vi "App - analyze RUS V6.vi"() -> ()   [LabVIEW 2015] (continued)
Field(T) "=0.0}, {"temperature"=205.505, "temperature str"="205.50500", "file path"=path "D:/Data/Ultrasound/LSCO/LSCO22__130814c/5_Cooling_2nd_try/September_2014/091614/205.50500K_500_2500_2.10000V_0.00000T_Sep16-2014__13-51-53_001_091614.bin", "last mod"=timestamp(3493734713 s since 1904-01-01), "file name str"="D:\\Data\\Ultrasound\\LSCO\\LSCO22__130814c\\5_Cooling_2nd_try\\September_2014\\091614\\205.50500K_500_2500_2.10000V_0.00000T_Sep16-2014__13-51-53_001_091614.bin", "mod time(min)"=58228911.88333333, "file format"=enum."binary", "power(V)"=2.1, "Magn Field(T) "=0.0}, {"temperature"=205.23, "temperature str"="205.23000", "file path"=path "D:/Data/Ultrasound/LSCO/LSCO22__130814c/5_Cooling_2nd_try/September_2014/091614/205.23000K_500_2500_2.10000V_0.00000T_Sep16-2014__13-53-13_001_091614.bin", "last mod"=timestamp(3493734793 s since 1904-01-01), "file name str"="D:\\Data\\Ultrasound\\LSCO\\LSCO22__130814c\\5_Cooling_2nd_try\\September_2014\\091614\\205.23000K_500_2500_2.10000V_0.00000T_Sep16-2014__13-53-13_001_091614.bin", "mod time(min)"=58228913.21666667, "file format"=enum."binary", "power(V)"=2.1, "Magn Field(T) "=0.0}, {"temperature"=204.949, "temperature str"="204.94900", "file path"=path "D:/Data/Ultrasound/LSCO/LSCO22__130814c/5_Cooling_2nd_try/September_2014/091614/204.94900K_500_2500_2.10000V_0.00000T_Sep16-2014__13-54-32_001_091614.bin", "last mod"=timestamp(3493734872 s since 1904-01-01), "file name str"="D:\\Data\\Ultrasound\\LSCO\\LSCO22__130814c\\5_Cooling_2nd_try\\September_2014\\091614\\204.94900K_500_2500_2.10000V_0.00000T_Sep16-2014__13-54-32_001_091614.bin", "mod time(min)"=58228914.53333333, "file format"=enum."binary", "power(V)"=2.1, "Magn Field(T) "=0.0}, {"temperature"=204.683, "temperature str"="204.68300", "file path"=path "D:/Data/Ultrasound/LSCO/LSCO22__130814c/5_Cooling_2nd_try/September_2014/091614/204.68300K_500_2500_2.10000V_0.00000T_Sep16-2014__13-55-52_001_091614.bin", "last mod"=timestamp(3493734952 s since 1904-01-01), "file name str"="D:\\Data\\Ultrasound\\LSCO\\LSCO22__130814c\\5_Cooling_2nd_try\\September_2014\\091614\\204.68300K_500_2500_2.10000V_0.00000T_Sep16-2014__13-55-52_001_091614.bin", "mod time(min)"=58228915.86666667, "file format"=enum."binary", "power(V)"=2.1, "Magn Field(T) "=0.0}, {"temperature"=204.406, "temperature str"="204.40600", "file path"=path "D:/Data/Ultrasound/LSCO/LSCO22__130814c/5_Cooling_2nd_try/September_2014/091614/204.40600K_500_2500_2.10000V_0.00000T_Sep16-2014__13-57-11_001_091614.bin", "last mod"=timestamp(3493735031 s since 1904-01-01), "file name str"="D:\\Data\\Ultrasound\\LSCO\\LSCO22__130814c\\5_Cooling_2nd_try\\September_2014\\091614\\204.40600K_500_2500_2.10000V_0.00000T_Sep16-2014__13-57-11_001_091614.bin", "mod time(min)"=58228917.18333333, "file format"=enum."binary", "power(V)"=2.1, "Magn Field(T) "=0.0}, {"temperature"=204.135, "temperature str"="204.13500", "file path"=path "D:/Data/Ultrasound/LSCO/LSCO22__130814c/5_Cooling_2nd_try/September_2014/091614/204.13500K_500_2500_2.10000V_0.00000T_Sep16-2014__13-58-30_001_091614.bin", "last mod"=timestamp(3493735110 s since 1904-01-01), "file name str"="D:\\Data\\Ultrasound\\LSCO\\LSCO22__130814c\\5_Cooling_2nd_try\\September_2014\\091614\\204.13500K_500_2500_2.10000V_0.00000T_Sep16-2014__13-58-30_001_091614.bin", "mod time(min)"=58228918.5, "file format"=enum."binary", "power(V)"=2.1, "Magn Field(T) "=0.0}, {"temperature"=203.855, "temperature str"="203.85500", "file path"=path "D:/Data/Ultrasound/LSCO/LSCO22__130814c/5_Cooling_2nd_try/September_2014/091614/203.85500K_500_2500_2.10000V_0.00000T_Sep16-2014__13-59-50_001_091614.bin", "last mod"=timestamp(3493735190 s since 1904-01-01), "file name str"="D:\\Data\\Ultrasound\\LSCO\\LSCO22__130814c\\5_Cooling_2nd_try\\September_2014\\091614\\203.85500K_500_2500_2.10000V_0.00000T_Sep16-2014__13-59-50_001_091614.bin", "mod time(min)"=58228919.833333336, "file format"=enum."binary", "power(V)"=2.1, "Magn Field(T) "=0.0}, {"temperature"=203.577, "temperature str"="203.57700", "file path"=path "D:/Data/Ultrasound/LSCO/LSCO22__130814c/5_Cooling_2nd_try/September_2014/091614/203.57700K_500_2500_2.10000V_0.00000T_Sep16-2014__14-01-09_001_091614.bin", "last mod"=timestamp(3493735269 s since 1904-01-01), "file name str"="D:\\Data\\Ultrasound\\LSCO\\LSCO22__130814c\\5_Cooling_2nd_try\\September_2014\\091614\\203.57700K_500_2500_2.10000V_0.00000T_Sep16-2014__14-01-09_001_091614.bin", "mod time(min)"=58228921.15, "file format"=enum."binary", "power(V)"=2.1, "Magn Field(T) "=0.0}, {"temperature"=203.306, "temperature str"="203.30600", "file path"=path "D:/Data/Ultrasound/LSCO/LSCO22__130814c/5_Cooling_2nd_try/September_2014/091614/203.30600K_500_2500_2.10000V_0.00000T_Sep16-2014__14-02-28_001_091614.bin", "last mod"=timestamp(3493735348 s since 1904-01-01), "file name str"="D:\\Data\\Ultrasound\\LSCO\\LSCO22__130814c\\5_Cooling_2nd_try\\September_2014\\091614\\203.30600K_500_2500_2.10000V_0.00000T_Sep16-2014__14-02-28_001_091614.bin", "mod time(min)"=58228922.46666667, "file format"=enum."binary", "power(V)"=2.1, "Magn Field(T) "=0.0}, {"temperature"=203.002, "temperature str"="203.00200", "file path"=path "D:/Data/Ultrasound/LSCO/LSCO22__130814c/5_Cooling_2nd_try/September_2014/091614/203.00200K_500_2500_2.10000V_0.00000T_Sep16-2014__14-03-54_001_091614.bin", "last mod"=timestamp(3493735434 s since 1904-01-01), "file name str"="D:\\Data\\Ultrasound\\LSCO\\LSCO22__130814c\\5_Cooling_2nd_try\\September_2014\\091614\\203.00200K_500_2500_2.10000V_0.00000T_Sep16-2014__14-03-54_001_091614.bin", "mod time(min)"=58228923.9, "file format"=enum."binary", "power(V)"=2.1, "Magn Field(T) "=0.0}, {"temperature"=202.734, "temperature str"="202.73400", "file path"=path "D:/Data/Ultrasound/LSCO/LSCO22__130814c/5_Cooling_2nd_try/September_2014/091614/202.73400K_500_2500_2.10000V_0.00000T_Sep16-2014__14-05-13_001_091614.bin", "last mod"=timestamp(3493735513 s since 1904-01-01), "file name str"="D:\\Data\\Ultrasound\\LSCO\\LSCO22__130814c\\5_Cooling_2nd_try\\September_2014\\091614\\202.73400K_500_2500_2.10000V_0.00000T_Sep16-2014__14-05-13_001_091614.bin", "mod time(min)"=58228925.21666667, "file format"=enum."binary", "power(V)"=2.1, "Magn Field(T) "=0.0}, {"temperature"=202.449, "temperature str"="202.44900", "file path"=path "D:/Data/Ultrasound/LSCO/LSCO22__130814c/5_Cooling_2nd_try/September_2014/091614/202.44900K_500_2500_2.10000V_0.00000T_Sep16-2014__14-06-32_001_091614.bin", "last mod"=timestamp(3493735592 s since 1904-01-01), "file name str"="D:\\Data\\Ultrasound\\LSCO\\LSCO22__130814c\\5_Cooling_2nd_try\\September_2014\\091614\\202.44900K_500_2500_2.10000V_0.00000T_Sep16-2014__14-06-32_001_091614.bin", "mod time(min)"=58228926.53333333, "file format"=enum."binary", "power(V)"=2.1, "Magn Field(T) "=0.0}, {"temperature"=202.176, "temperature str"="202.17600", "file path"=path "D:/Data/Ultrasound/LSCO/LSCO22__130814c/5_Cooling_2nd_try/September_2014/091614/202.17600K_500_2500_2.10000V_0.00000T_Sep16-2014__14-07-52_001_091614.bin", "last mod"=timestamp(3493735672 s since 1904-01-01), "file name str"="D:\\Data\\Ultrasound\\LSCO\\LSCO22__130814c\\5_Cooling_2nd_try\\September_2014\\091614\\202.17600K_500_2500_2.10000V_0.00000T_Sep16-2014__14-07-52_001_091614.bin", "mod time(min)"=58228927.86666667, "file format"=enum."binary", "power(V)"=2.1, "Magn Field(T) "=0.0}, {"temperature"=201.892, "temperature str"="201.89200", "file path"=path "D:/Data/Ultrasound/LSCO/LSCO22__130814c/5_Cooling_2nd_try/September_2014/091614/201.89200K_500_2500_2.10000V_0.00000T_Sep16-2014__14-09-11_001_091614.bin", "last mod"=timestamp(3493735751 s since 1904-01-01), "file name str"="D:\\Data\\Ultrasound\\LSCO\\LSCO22__130814c\\5_Cooling_2nd_try\\September_2014\\091614\\201.89200K_500_2500_2.10000V_0.00000T_Sep16-2014__14-09-11_001_091614.bin", "mod time(min)"=58228929.18333333, "file format"=enum."binary", "power(V)"=2.1, "Magn Field(T) "=0.0}, {"temperature"=201.608, "temperature str"="201.60800", "file path"=path "D:/Data/Ultrasound/LSCO/LSCO22__130814c/5_Cooling_2nd_try/September_2014/091614/201.60800K_500_2500_2.10000V_0.00000T_Sep16-2014__14-10-30_001_091614.bin", "last mod"=timestamp(3493735830 s since 1904-01-01), "file name str"="D:\\Data\\Ultrasound\\LSCO\\LSCO22__130814c\\5_Cooling_2nd_try\\September_2014\\091614\\201.60800K_500_2500_2.10000V_0.00000T_Sep16-2014__14-10-30_001_091614.bin", "mod time(min)"=58228930.5, "file format"=enum."binary", "power(V)"=2.1, "Magn Field(T) "=0.0}, {"temperature"=201.335, "temperature str"="201.33500", "file path"=path "D:/Data/Ultrasound/LSCO/LSCO22__130814c/5_Cooling_2nd_try/September_2014/091614/201.33500K_500_2500_2.10000V_0.00000T_Sep16-2014__14-11-50_001_091614.bin", "last mod"=timestamp(3493735910 s since 1904-01-01), "file name str"="D:\\Data\\Ultrasound\\LSCO\\LSCO22__130814c\\5_Cooling_2nd_try\\September_2014\\091614\\201.33500K_500_2500_2.10000V_0.00000T_Sep16-2014__14-11-50_001_091614.bin", "mod time(min)"=58228931.833333336, "file format"=enum."binary", "power(V)"=2.1, "Magn Field(T) "=0.0}, {"temperature"=201.049, "temperature str"="201.04900", "file path"=path "D:/Data/Ultrasound/LSCO/LSCO22__130814c/5_Cooling_2nd_try/September_2014/091614/201.04900K_500_2500_2.10000V_0.00000T_Sep16-2014__14-13-09_001_091614.bin", "last mod"=timestamp(3493735989 s since 1904-01-01), "file name str"="D:\\Data\\Ultrasound\\LSCO\\LSCO22__130814c\\5_Cooling_2nd_try\\September_2014\\091614\\201.04900K_500_2500_2.10000V_0.00000T_Sep16-2014__14-13-09_001_091614.bin", "mod time(min)"=58228933.15, "file format"=enum."binary", "power(V)"=2.1, "Magn Field(T) "=0.0}, {"temperature"=200.772, "temperature str"="200.77200", "file path"=path "D:/Data/Ultrasound/LSCO/LSCO22__130814c/5_Cooling_2nd_try/September_2014/091614/200.77200K_500_2500_2.10000V_0.00000T_Sep16-2014__14-14-29_001_091614.bin", "last mod"=timestamp(3493736069 s since 1904-01-01), "file name str"="D:\\Data\\Ultrasound\\LSCO\\LSCO22__130814c\\5_Cooling_2nd_try\\September_2014\\091614\\200.77200K_500_2500_2.10000V_0.00000T_Sep16-2014__14-14-29_001_091614.bin", "mod time(min)"=58228934.483333334, "file format"=enum."binary", "power(V)"=2.1, "Magn Field(T) "=0.0}, {"temperature"=200.485, "temperature str"="200.48500", "file path"=path "D:/Data/Ultrasound/LSCO/LSCO22__130814c/5_Cooling_2nd_try/September_2014/091614/200.48500K_500_2500_2.10000V_0.00000T_Sep16-2014__14-15-48_001_091614.bin", "last mod"=timestamp(3493736148 s since 1904-01-01), "file name str"="D:\\Data\\Ultrasound\\LSCO\\LSCO22__130814c\\5_Cooling_2nd_try\\September_2014\\091614\\200.48500K_500_2500_2.10000V_0.00000T_Sep16-2014__14-15-48_001_091614.bin", "mod time(min)"=58228935.8, "file format"=enum."binary", "power(V)"=2.1, "Magn Field(T) "=0.0}, {"temperature"=200.196, "temperature str"="200.19600", "file path"=path "D:/Data/Ultrasound/LSCO/LSCO22__130814c/5_Cooling_2nd_try/September_2014/091614/200.19600K_500_2500_2.10000V_0.00000T_Sep16-2014__14-17-07_001_091614.bin", "last mod"=timestamp(3493736227 s since 1904-01-01), "file name str"="D:\\Data\\Ultrasound\\LSCO\\LSCO22__130814c\\5_Cooling_2nd_try\\September_2014\\091614\\200.19600K_500_2500_2.10000V_0.00000T_Sep16-2014__14-17-07_001_091614.bin", "mod time(min)"=58228937.11666667, "file format"=enum."binary", "power(V)"=2.1, "Magn Field(T) "=0.0}, {"temperature"=199.92, "temperature str"="199.92000", "file path"=path "D:/Data/Ultrasound/LSCO/LSCO22__130814c/5_Cooling_2nd_try/September_2014/091614/199.92000K_500_2500_2.10000V_0.00000T_Sep16-2014__14-18-27_001_091614.bin", "last mod"=timestamp(3493736307 s since 1904-01-01), "file name str"="D:\\Data\\Ultrasound\\LSCO\\LSCO22__130814c\\5_Cooling_2nd_try\\September_2014\\091614\\199.92000K_500_2500_2.10000V_0.00000T_Sep16-2014__14-18-27_001_091614.bin", "mod time(min)"=58228938.45, "file format"=enum."binary", "power(V)"=2.1, "Magn Field(T) "=0.0}, {"temperature"=199.633, "temperature str"="199.63300", "file path"=path "D:/Data/Ultrasound/LSCO/LSCO22__130814c/5_Cooling_2nd_try/September_2014/091614/199.63300K_500_2500_2.10000V_0.00000T_Sep16-2014__14-19-46_001_091614.bin", "last mod"=timestamp(3493736386 s since 1904-01-01), "file name str"="D:\\Data\\Ultrasound\\LSCO\\LSCO22__130814c\\5_Cooling_2nd_try\\September_2014\\091614\\199.63300K_500_2500_2.10000V_0.00000T_Sep16-2014__14-19-46_001_091614.bin", "mod time(min)"=58228939.766666666, "file format"=enum."binary", "power(V)"=2.1, "Magn Field(T) "=0.0}, {"temperature"=199.352, "temperature str"="199.35200", "file path"=path "D:/Data/Ultrasound/LSCO/LSCO22__130814c/5_Cooling_2nd_try/September_2014/091614/199.35200K_500_2500_2.10000V_0.00000T_Sep16-2014__14-21-05_001_091614.bin", "last mod"=timestamp(3493736465 s since 1904-01-01), "file name str"="D:\\Data\\Ultrasound\\LSCO\\LSCO22__130814c\\5_Cooling_2nd_try\\September_2014\\091614\\199.35200K_500_2500_2.10000V_0.00000T_Sep16-2014__14-21-05_001_091614.bin", "mod time(min)"=58228941.083333336, "file format"=enum."binary", "power(V)"=2.1, "Magn Field(T) "=0.0}, {"temperature"=199.061, "temperature str"="199.06100", "file path"=path "D:/Data/Ultrasound/LSCO/LSCO22__130814c/5_Cooling_2nd_try/September_2014/091614/199.06100K_500_2500_2.10000V_0.00000T_Sep16-2014__14-22-25_001_091614.bin", "last mod"=timestamp(3493736545 s since 1904-01-01), "file name str"="D:\\Data\\Ultrasound\\LSCO\\LSCO22__130814c\\5_Cooling_2nd_try\\September_2014\\091614\\199.06100K_500_2500_2.10000V_0.00000T_Sep16-2014__14-22-25_001_091614.bin", "mod time(min)"=58228942.416666664, "file format"=enum."binary", "power(V)"=2.1, "Magn Field(T) "=0.0}, {"temperature"=198.769, "temperature str"="198.76900", "file path"=path "D:/Data/Ultrasound/LSCO/LSCO22__130814c/5_Cooling_2nd_try/September_2014/091614/198.76900K_500_2500_2.10000V_0.00000T_Sep16-2014__14-23-44_001_091614.bin", "last mod"=timestamp(3493736624 s since 1904-01-01), "file name str"="D:\\Data\\Ultrasound\\LSCO\\LSCO22__130814c\\5_Cooling_2nd_try\\September_2014\\091614\\198.76900K_500_2500_2.10000V_0.00000T_Sep16-2014__14-23-44_001_091614.bin", "mod time(min)"=58228943.733333334, "file format"=enum."binary", "power(V)"=2.1, "Magn Field(T) "=0.0}, {"temperature"=198.49, "temperature str"="198.49000", "file path"=path "D:/Data/Ultrasound/LSCO/LSCO22__130814c/5_Cooling_2nd_try/September_2014/091614/198.49000K_500_2500_2.10000V_0.00000T_Sep16-2014__14-25-04_001_091614.bin", "last mod"=timestamp(3493736704 s since 1904-01-01), "file name str"="D:\\Data\\Ultrasound\\LSCO\\LSCO22__130814c\\5_Cooling_2nd_try\\September_2014\\091614\\198.49000K_500_2500_2.10000V_0.00000T_Sep16-2014__14-25-04_001_091614.bin", "mod time(min)"=58228945.06666667, "file format"=enum."binary", "power(V)"=2.1, "Magn Field(T) "=0.0}, {"temperature"=198.198, "temperature str"="198.19800", "file path"=path "D:/Data/Ultrasound/LSCO/LSCO22__130814c/5_Cooling_2nd_try/September_2014/091614/198.19800K_500_2500_2.10000V_0.00000T_Sep16-2014__14-26-23_001_091614.bin", "last mod"=timestamp(3493736783 s since 1904-01-01), "file name str"="D:\\Data\\Ultrasound\\LSCO\\LSCO22__130814c\\5_Cooling_2nd_try\\September_2014\\091614\\198.19800K_500_2500_2.10000V_0.00000T_Sep16-2014__14-26-23_001_091614.bin", "mod time(min)"=58228946.38333333, "file format"=enum."binary", "power(V)"=2.1, "Magn Field(T) "=0.0}, {"temperature"=197.916, "temperature str"="197.91600", "file path"=path "D:/Data/Ultrasound/LSCO/LSCO22__130814c/5_Cooling_2nd_try/September_2014/091614/197.91600K_500_2500_2.10000V_0.00000T_Sep16-2014__14-27-42_001_091614.bin", "last mod"=timestamp(3493736862 s since 1904-01-01), "file name str"="D:\\Data\\Ultrasound\\LSCO\\LSCO22__130814c\\5_Cooling_2nd_try\\September_2014\\091614\\197.91600K_500_2500_2.10000V_0.00000T_Sep16-2014__14-27-42_001_091614.bin", "mod time(min)"=58228947.7, "file format"=enum."binary", "power(V)"=2.1, "Magn Field(T) "=0.0}, {"temperature"=197.62, "temperature str"="197.62000", "file path"=path "D:/Data/Ultrasound/LSCO/LSCO22__130814c/5_Cooling_2nd_try/September_2014/091614/197.62000K_500_2500_2.10000V_0.00000T_Sep16-2014__14-29-02_001_091614.bin", "last mod"=timestamp(3493736942 s since 1904-01-01), "file name str"="D:\\Data\\Ultrasound\\LSCO\\LSCO22__130814c\\5_Cooling_2nd_try\\September_2014\\091614\\197.62000K_500_2500_2.10000V_0.00000T_Sep16-2014__14-29-02_001_091614.bin", "mod time(min)"=58228949.03333333, "file format"=enum."binary", "power(V)"=2.1, "Magn Field(T) "=0.0}, {"temperature"=197.325, "temperature str"="197.32500", "file path"=path "D:/Data/Ultrasound/LSCO/LSCO22__130814c/5_Cooling_2nd_try/September_2014/091614/197.32500K_500_2500_2.10000V_0.00000T_Sep16-2014__14-30-21_001_091614.bin", "last mod"=timestamp(3493737021 s since 1904-01-01), "file name str"="D:\\Data\\Ultrasound\\LSCO\\LSCO22__130814c\\5_Cooling_2nd_try\\September_2014\\091614\\197.32500K_500_2500_2.10000V_0.00000T_Sep16-2014__14-30-21_001_091614.bin", "mod time(min)"=58228950.35, "file format"=enum."binary", "power(V)"=2.1, "Magn Field(T) "=0.0}, {"temperature"=197.042, "temperature str"="197.04200", "file path"=path "D:/Data/Ultrasound/LSCO/LSCO22__130814c/5_Cooling_2nd_try/September_2014/091614/197.04200K_500_2500_2.10000V_0.00000T_Sep16-2014__14-31-40_001_091614.bin", "last mod"=timestamp(3493737100 s since 1904-01-01), "file name str"="D:\\Data\\Ultrasound\\LSCO\\LSCO22__130814c\\5_Cooling_2nd_try\\September_2014\\091614\\197.04200K_500_2500_2.10000V_0.00000T_Sep16-2014__14-31-40_001_091614.bin", "mod time(min)"=58228951.666666664, "file format"=enum."binary", "power(V)"=2.1, "Magn Field(T) "=0.0}, {"temperature"=196.746, "temperature str"="196.74600", "file path"=path "D:/Data/Ultrasound/LSCO/LSCO22__130814c/5_Cooling_2nd_try/September_2014/091614/196.74600K_500_2500_2.10000V_0.00000T_Sep16-2014__14-33-00_001_091614.bin", "last mod"=timestamp(3493737180 s since 1904-01-01), "file name str"="D:\\Data\\Ultrasound\\LSCO\\LSCO22__130814c\\5_Cooling_2nd_try\\September_2014\\091614\\196.74600K_500_2500_2.10000V_0.00000T_Sep16-2014__14-33-00_001_091614.bin", "mod time(min)"=58228953.0, "file format"=enum."binary", "power(V)"=2.1, "Magn Field(T) "=0.0}, {"temperature"=196.459, "temperature str"="196.45900", "file path"=path "D:/Data/Ultrasound/LSCO/LSCO22__130814c/5_Cooling_2nd_try/September_2014/091614/196.45900K_500_2500_2.10000V_0.00000T_Sep16-2014__14-34-19_001_091614.bin", "last mod"=timestamp(3493737259 s since 1904-01-01), "file name str"="D:\\Data\\Ultrasound\\LSCO\\LSCO22__130814c\\5_Cooling_2nd_try\\September_2014\\091614\\196.45900K_500_2500_2.10000V_0.00000T_Sep16-2014__14-34-19_001_091614.bin", "mod time(min)"=58228954.31666667, "file format"=enum."binary", "power(V)"=2.1, "Magn Field(T) "=0.0}, {"temperature"=196.161, "temperature str"="196.16100", "file path"=path "D:/Data/Ultrasound/LSCO/LSCO22__130814c/5_Cooling_2nd_try/September_2014/091614/196.16100K_500_2500_2.10000V_0.00000T_Sep16-2014__14-35-39_001_091614.bin", "last mod"=timestamp(3493737339 s since 1904-01-01), "file name str"="D:\\Data\\Ultrasound\\LSCO\\LSCO22__130814c\\5_Cooling_2nd_try\\September_2014\\091614\\196.16100K_500_2500_2.10000V_0.00000T_Sep16-2014__14-35-39_001_091614.bin", "mod time(min)"=58228955.65, "file format"=enum."binary", "power(V)"=2.1, "Magn Field(T) "=0.0}, {"temperature"=195.862, "temperature str"="195.86200", "file path"=path "D:/Data/Ultrasound/LSCO/LSCO22__130814c/5_Cooling_2nd_try/September_2014/091614/195.86200K_500_2500_2.10000V_0.00000T_Sep16-2014__14-36-58_001_091614.bin", "last mod"=timestamp(3493737418 s since 1904-01-01), "file name str"="D:\\Data\\Ultrasound\\LSCO\\LSCO22__130814c\\5_Cooling_2nd_try\\September_2014\\091614\\195.86200K_500_2500_2.10000V_0.00000T_Sep16-2014__14-36-58_001_091614.bin", "mod time(min)"=58228956.96666667, "file format"=enum."binary", "power(V)"=2.1, "Magn Field(T) "=0.0}, {"temperature"=195.573, "temperature str"="195.57300", "file path"=path "D:/Data/Ultrasound/LSCO/LSCO22__130814c/5_Cooling_2nd_try/September_2014/091614/195.57300K_500_2500_2.10000V_0.00000T_Sep16-2014__14-38-17_001_091614.bin", "last mod"=timestamp(3493737497 s since 1904-01-01), "file name str"="D:\\Data\\Ultrasound\\LSCO\\LSCO22__130814c\\5_Cooling_2nd_try\\September_2014\\091614\\195.57300K_500_2500_2.10000V_0.00000T_Sep16-2014__14-38-17_001_091614.bin", "mod time(min)"=58228958.28333333, "file format"=enum."binary", "power(V)"=2.1, "Magn Field(T) "=0.0}, {"temperature"=195.277, "temperature str"="195.27700", "file path"=path "D:/Data/Ultrasound/LSCO/LSCO22__130814c/5_Cooling_2nd_try/September_2014/091614/195.27700K_500_2500_2.10000V_0.00000T_Sep16-2014__14-39-37_001_091614.bin", "last mod"=timestamp(3493737577 s since 1904-01-01), "file name str"="D:\\Data\\Ultrasound\\LSCO\\LSCO22__130814c\\5_Cooling_2nd_try\\September_2014\\091614\\195.27700K_500_2500_2.10000V_0.00000T_Sep16-2014__14-39-37_001_091614.bin", "mod time(min)"=58228959.61666667, "file format"=enum."binary", "power(V)"=2.1, "Magn Field(T) "=0.0}, {"temperature"=194.992, "temperature str"="194.99200", "file path"=path "D:/Data/Ultrasound/LSCO/LSCO22__130814c/5_Cooling_2nd_try/September_2014/091614/194.99200K_500_2500_2.10000V_0.00000T_Sep16-2014__14-40-56_001_091614.bin", "last mod"=timestamp(3493737656 s since 1904-01-01), "file name str"="D:\\Data\\Ultrasound\\LSCO\\LSCO22__130814c\\5_Cooling_2nd_try\\September_2014\\091614\\194.99200K_500_2500_2.10000V_0.00000T_Sep16-2014__14-40-56_001_091614.bin", "mod time(min)"=58228960.93333333, "file format"=enum."binary", "power(V)"=2.1, "Magn Field(T) "=0.0}, {"temperature"=194.69, "temperature str"="194.69000", "file path"=path "D:/Data/Ultrasound/LSCO/LSCO22__130814c/5_Cooling_2nd_try/September_2014/091614/194.69000K_500_2500_2.10000V_0.00000T_Sep16-2014__14-42-15_001_091614.bin", "last mod"=timestamp(3493737735 s since 1904-01-01), "file name str"="D:\\Data\\Ultrasound\\LSCO\\LSCO22__130814c\\5_Cooling_2nd_try\\September_2014\\091614\\194.69000K_500_2500_2.10000V_0.00000T_Sep16-2014__14-42-15_001_091614.bin", "mod time(min)"=58228962.25, "file format"=enum."binary", "power(V)"=2.1, "Magn Field(T) "=0.0}, {"temperature"=194.386, "temperature str"="194.38600", "file path"=path "D:/Data/Ultrasound/LSCO/LSCO22__130814c/5_Cooling_2nd_try/September_2014/091614/194.38600K_500_2500_2.10000V_0.00000T_Sep16-2014__14-43-35_001_091614.bin", "last mod"=timestamp(3493737815 s since 1904-01-01), "file name str"="D:\\Data\\Ultrasound\\LSCO\\LSCO22__130814c\\5_Cooling_2nd_try\\September_2014\\091614\\194.38600K_500_2500_2.10000V_0.00000T_Sep16-2014__14-43-35_001_091614.bin", "mod time(min)"=58228963.583333336, "file format"=enum."binary", "power(V)"=2.1, "Magn Field(T) "=0.0}, {"temperature"=194.091, "temperature str"="194.09100", "file path"=path "D:/Data/Ultrasound/LSCO/LSCO22__130814c/5_Cooling_2nd_try/September_2014/091614/194.09100K_500_2500_2.10000V_0.00000T_Sep16-2014__14-44-54_001_091614.bin", "last mod"=timestamp(3493737894 s since 1904-01-01), "file name str"="D:\\Data\\Ultrasound\\LSCO\\LSCO22__130814c\\5_Cooling_2nd_try\\September_2014\\091614\\194.09100K_500_2500_2.10000V_0.00000T_Sep16-2014__14-44-54_001_091614.bin", "mod time(min)"=58228964.9, "file format"=enum."binary", "power(V)"=2.1, "Magn Field(T) "=0.0}, {"temperature"=193.788, "temperature str"="193.78800", "file path"=path "D:/Data/Ultrasound/LSCO/LSCO22__130814c/5_Cooling_2nd_try/September_2014/091614/193.78800K_500_2500_2.10000V_0.00000T_Sep16-2014__14-46-13_001_091614.bin", "last mod"=timestamp(3493737973 s since 1904-01-01), "file name str"="D:\\Data\\Ultrasound\\LSCO\\LSCO22__130814c\\5_Cooling_2nd_try\\September_2014\\091614\\193.78800K_500_2500_2.10000V_0.00000T_Sep16-2014__14-46-13_001_091614.bin", "mod time(min)"=58228966.21666667, "file format"=enum."binary", "power(V)"=2.1, "Magn Field(T) "=0.0}, {"temperature"=193.485, "temperature str"="193.48500", "file path"=path "D:/Data/Ultrasound/LSCO/LSCO22__130814c/5_Cooling_2nd_try/September_2014/091614/193.48500K_500_2500_2.10000V_0.00000T_Sep16-2014__14-47-33_001_091614.bin", "last mod"=timestamp(3493738053 s since 1904-01-01), "file name str"="D:\\Data\\Ultrasound\\LSCO\\LSCO22__130814c\\5_Cooling_2nd_try\\September_2014\\091614\\193.48500K_500_2500_2.10000V_0.00000T_Sep16-2014__14-47-33_001_091614.bin", "mod time(min)"=58228967.55, "file format"=enum."binary", "power(V)"=2.1, "Magn Field(T) "=0.0}, {"temperature"=193.192, "temperature str"="193.19200", "file path"=path "D:/Data/Ultrasound/LSCO/LSCO22__130814c/5_Cooling_2nd_try/September_2014/091614/193.19200K_500_2500_2.10000V_0.00000T_Sep16-2014__14-48-52_001_091614.bin", "last mod"=timestamp(3493738132 s since 1904-01-01), "file name str"="D:\\Data\\Ultrasound\\LSCO\\LSCO22__130814c\\5_Cooling_2nd_try\\September_2014\\091614\\193.19200K_500_2500_2.10000V_0.00000T_Sep16-2014__14-48-52_001_091614.bin", "mod time(min)"=58228968.86666667, "file format"=enum."binary", "power(V)"=2.1, "Magn Field(T) "=0.0}, {"temperature"=192.887, "temperature str"="192.88700", "file path"=path "D:/Data/Ultrasound/LSCO/LSCO22__130814c/5_Cooling_2nd_try/September_2014/091614/192.88700K_500_2500_2.10000V_0.00000T_Sep16-2014__14-50-12_001_091614.bin", "last mod"=timestamp(3493738212 s since 1904-01-01), "file name str"="D:\\Data\\Ultrasound\\LSCO\\LSCO22__130814c\\5_Cooling_2nd_try\\September_2014\\091614\\192.88700K_500_2500_2.10000V_0.00000T_Sep16-2014__14-50-12_001_091614.bin", "mod time(min)"=58228970.2, "file format"=enum."binary", "power(V)"=2.1, "Magn Field(T) "=0.0}, {"temperature"=192.594, "temperature str"="192.59400", "file path"=path "D:/Data/Ultrasound/LSCO/LSCO22__130814c/5_Cooling_2nd_try/September_2014/091614/192.59400K_500_2500_2.10000V_0.00000T_Sep16-2014__14-51-31_001_091614.bin", "last mod"=timestamp(3493738291 s since 1904-01-01), "file name str"="D:\\Data\\Ultrasound\\LSCO\\LSCO22__130814c\\5_Cooling_2nd_try\\September_2014\\091614\\192.59400K_500_2500_2.10000V_0.00000T_Sep16-2014__14-51-31_001_091614.bin", "mod time(min)"=58228971.516666666, "file format"=enum."binary", "power(V)"=2.1, "Magn Field(T) "=0.0}, {"temperature"=192.288, "temperature str"="192.28800", "file path"=path "D:/Data/Ultrasound/LSCO/LSCO22__130814c/5_Cooling_2nd_try/September_2014/091614/192.28800K_500_2500_2.10000V_0.00000T_Sep16-2014__14-52-50_001_091614.bin", "last mod"=timestamp(3493738370 s since 1904-01-01), "file name str"="D:\\Data\\Ultrasound\\LSCO\\LSCO22__130814c\\5_Cooling_2nd_try\\September_2014\\091614\\192.28800K_500_2500_2.10000V_0.00000T_Sep16-2014__14-52-50_001_091614.bin", "mod time(min)"=58228972.833333336, "file format"=enum."binary", "power(V)"=2.1, "Magn Field(T) "=0.0}, {"temperature"=191.978, "temperature str"="191.97800", "file path"=path "D:/Data/Ultrasound/LSCO/LSCO22__130814c/5_Cooling_2nd_try/September_2014/091614/191.97800K_500_2500_2.10000V_0.00000T_Sep16-2014__14-54-10_001_091614.bin", "last mod"=timestamp(3493738450 s since 1904-01-01), "file name str"="D:\\Data\\Ultrasound\\LSCO\\LSCO22__130814c\\5_Cooling_2nd_try\\September_2014\\091614\\191.97800K_500_2500_2.10000V_0.00000T_Sep16-2014__14-54-10_001_091614.bin", "mod time(min)"=58228974.166666664, "file format"=enum."binary", "power(V)"=2.1, "Magn Field(T) "=0.0}, {"temperature"=191.681, "temperature str"="191.68100", "file path"=path "D:/Data/Ultrasound/LSCO/LSCO22__130814c/5_Cooling_2nd_try/September_2014/091614/191.68100K_500_2500_2.10000V_0.00000T_Sep16-2014__14-55-29_001_091614.bin", "last mod"=timestamp(3493738529 s since 1904-01-01), "file name str"="D:\\Data\\Ultrasound\\LSCO\\LSCO22__130814c\\5_Cooling_2nd_try\\September_2014\\091614\\191.68100K_500_2500_2.10000V_0.00000T_Sep16-2014__14-55-29_001_091614.bin", "mod time(min)"=58228975.483333334, "file format"=enum."binary", "power(V)"=2.1, "Magn Field(T) "=0.0}, {"temperature"=191.372, "temperature str"="191.37200", "file path"=path "D:/Data/Ultrasound/LSCO/LSCO22__130814c/5_Cooling_2nd_try/September_2014/091614/191.37200K_500_2500_2.10000V_0.00000T_Sep16-2014__14-56-48_001_091614.bin", "last mod"=timestamp(3493738608 s since 1904-01-01), "file name str"="D:\\Data\\Ultrasound\\LSCO\\LSCO22__130814c\\5_Cooling_2nd_try\\September_2014\\091614\\191.37200K_500_2500_2.10000V_0.00000T_Sep16-2014__14-56-48_001_091614.bin", "mod time(min)"=58228976.8, "file format"=enum."binary", "power(V)"=2.1, "Magn Field(T) "=0.0}, {"temperature"=191.076, "temperature str"="191.07600", "file path"=path "D:/Data/Ultrasound/LSCO/LSCO22__130814c/5_Cooling_2nd_try/September_2014/091614/191.07600K_500_2500_2.10000V_0.00000T_Sep16-2014__14-58-08_001_091614.bin", "last mod"=timestamp(3493738688 s since 1904-01-01), "file name str"="D:\\Data\\Ultrasound\\LSCO\\LSCO22__130814c\\5_Cooling_2nd_try\\September_2014\\091614\\191.07600K_500_2500_2.10000V_0.00000T_Sep16-2014__14-58-08_001_091614.bin", "mod time(min)"=58228978.13333333, "file format"=enum."binary", "power(V)"=2.1, "Magn Field(T) "=0.0}, {"temperature"=190.764, "temperature str"="190.76400", "file path"=path "D:/Data/Ultrasound/LSCO/LSCO22__130814c/5_Cooling_2nd_try/September_2014/091614/190.76400K_500_2500_2.10000V_0.00000T_Sep16-2014__14-59-27_001_091614.bin", "last mod"=timestamp(3493738767 s since 1904-01-01), "file name str"="D:\\Data\\Ultrasound\\LSCO\\LSCO22__130814c\\5_Cooling_2nd_try\\September_2014\\091614\\190.76400K_500_2500_2.10000V_0.00000T_Sep16-2014__14-59-27_001_091614.bin", "mod time(min)"=58228979.45, "file format"=enum."binary", "power(V)"=2.1, "Magn Field(T) "=0.0}, {"temperature"=190.453, "temperature str"="190.45300", "file path"=path "D:/Data/Ultrasound/LSCO/LSCO22__130814c/5_Cooling_2nd_try/September_2014/091614/190.45300K_500_2500_2.10000V_0.00000T_Sep16-2014__15-00-47_001_091614.bin", "last mod"=timestamp(3493738847 s since 1904-01-01), "file name str"="D:\\Data\\Ultrasound\\LSCO\\LSCO22__130814c\\5_Cooling_2nd_try\\September_2014\\091614\\190.45300K_500_2500_2.10000V_0.00000T_Sep16-2014__15-00-47_001_091614.bin", "mod time(min)"=58228980.78333333, "file format"=enum."binary", "power(V)"=2.1, "Magn Field(T) "=0.0}, {"temperature"=190.152, "temperature str"="190.15200", "file path"=path "D:/Data/Ultrasound/LSCO/LSCO22__130814c/5_Cooling_2nd_try/September_2014/091614/190.15200K_500_2500_2.10000V_0.00000T_Sep16-2014__15-02-06_001_091614.bin", "last mod"=timestamp(3493738926 s since 1904-01-01), "file name str"="D:\\Data\\Ultrasound\\LSCO\\LSCO22__130814c\\5_Cooling_2nd_try\\September_2014\\091614\\190.15200K_500_2500_2.10000V_0.00000T_Sep16-2014__15-02-06_001_091614.bin", "mod time(min)"=58228982.1, "file format"=enum."binary", "power(V)"=2.1, "Magn Field(T) "=0.0}, {"temperature"=189.843, "temperature str"="189.84300", "file path"=path "D:/Data/Ultrasound/LSCO/LSCO22__130814c/5_Cooling_2nd_try/September_2014/091614/189.84300K_500_2500_2.10000V_0.00000T_Sep16-2014__15-03-25_001_091614.bin", "last mod"=timestamp(3493739005 s since 1904-01-01), "file name str"="D:\\Data\\Ultrasound\\LSCO\\LSCO22__130814c\\5_Cooling_2nd_try\\September_2014\\091614\\189.84300K_500_2500_2.10000V_0.00000T_Sep16-2014__15-03-25_001_091614.bin", "mod time(min)"=58228983.416666664, "file format"=enum."binary", "power(V)"=2.1, "Magn Field(T) "=0.0}, {"temperature"=189.545, "temperature str"="189.54500", "file path"=path "D:/Data/Ultrasound/LSCO/LSCO22__130814c/5_Cooling_2nd_try/September_2014/091614/189.54500K_500_2500_2.10000V_0.00000T_Sep16-2014__15-04-45_001_091614.bin", "last mod"=timestamp(3493739085 s since 1904-01-01), "file name str"="D:\\Data\\Ultrasound\\LSCO\\LSCO22__130814c\\5_Cooling_2nd_try\\September_2014\\091614\\189.54500K_500_2500_2.10000V_0.00000T_Sep16-2014__15-04-45_001_091614.bin", "mod time(min)"=58228984.75, "file format"=enum."binary", "power(V)"=2.1, "Magn Field(T) "=0.0}, {"temperature"=189.231, "temperature str"="189.23100", "file path"=path "D:/Data/Ultrasound/LSCO/LSCO22__130814c/5_Cooling_2nd_try/September_2014/091614/189.23100K_500_2500_2.10000V_0.00000T_Sep16-2014__15-06-04_001_091614.bin", "last mod"=timestamp(3493739164 s since 1904-01-01), "file name str"="D:\\Data\\Ultrasound\\LSCO\\LSCO22__130814c\\5_Cooling_2nd_try\\September_2014\\091614\\189.23100K_500_2500_2.10000V_0.00000T_Sep16-2014__15-06-04_001_091614.bin", "mod time(min)"=58228986.06666667, "file format"=enum."binary", "power(V)"=2.1, "Magn Field(T) "=0.0}, {"temperature"=188.914, "temperature str"="188.91400", "file path"=path "D:/Data/Ultrasound/LSCO/LSCO22__130814c/5_Cooling_2nd_try/September_2014/091614/188.91400K_500_2500_2.10000V_0.00000T_Sep16-2014__15-07-23_001_091614.bin", "last mod"=timestamp(3493739243 s since 1904-01-01), "file name str"="D:\\Data\\Ultrasound\\LSCO\\LSCO22__130814c\\5_Cooling_2nd_try\\September_2014\\091614\\188.91400K_500_2500_2.10000V_0.00000T_Sep16-2014__15-07-23_001_091614.bin", "mod time(min)"=58228987.38333333, "file format"=enum."binary", "power(V)"=2.1, "Magn Field(T) "=0.0}, {"temperature"=188.611, "temperature str"="188.61100", "file path"=path "D:/Data/Ultrasound/LSCO/LSCO22__130814c/5_Cooling_2nd_try/September_2014/091614/188.61100K_500_2500_2.10000V_0.00000T_Sep16-2014__15-08-43_001_091614.bin", "last mod"=timestamp(3493739323 s since 1904-01-01), "file name str"="D:\\Data\\Ultrasound\\LSCO\\LSCO22__130814c\\5_Cooling_2nd_try\\September_2014\\091614\\188.61100K_500_2500_2.10000V_0.00000T_Sep16-2014__15-08-43_001_091614.bin", "mod time(min)"=58228988.71666667, "file format"=enum."binary", "power(V)"=2.1, "Magn Field(T) "=0.0}, {"temperature"=188.296, "temperature str"="188.29600", "file path"=path "D:/Data/Ultrasound/LSCO/LSCO22__130814c/5_Cooling_2nd_try/September_2014/091614/188.29600K_500_2500_2.10000V_0.00000T_Sep16-2014__15-10-02_001_091614.bin", "last mod"=timestamp(3493739402 s since 1904-01-01), "file name str"="D:\\Data\\Ultrasound\\LSCO\\LSCO22__130814c\\5_Cooling_2nd_try\\September_2014\\091614\\188.29600K_500_2500_2.10000V_0.00000T_Sep16-2014__15-10-02_001_091614.bin", "mod time(min)"=58228990.03333333, "file format"=enum."binary", "power(V)"=2.1, "Magn Field(T) "=0.0}, {"temperature"=187.992, "temperature str"="187.99200", "file path"=path "D:/Data/Ultrasound/LSCO/LSCO22__130814c/5_Cooling_2nd_try/September_2014/091614/187.99200K_500_2500_2.10000V_0.00000T_Sep16-2014__15-11-22_001_091614.bin", "last mod"=timestamp(3493739482 s since 1904-01-01), "file name str"="D:\\Data\\Ultrasound\\LSCO\\LSCO22__130814c\\5_Cooling_2nd_try\\September_2014\\091614\\187.99200K_500_2500_2.10000V_0.00000T_Sep16-2014__15-11-22_001_091614.bin", "mod time(min)"=58228991.36666667, "file format"=enum."binary", "power(V)"=2.1, "Magn Field(T) "=0.0}, {"temperature"=187.678, "temperature str"="187.67800", "file path"=path "D:/Data/Ultrasound/LSCO/LSCO22__130814c/5_Cooling_2nd_try/September_2014/091614/187.67800K_500_2500_2.10000V_0.00000T_Sep16-2014__15-12-41_001_091614.bin", "last mod"=timestamp(3493739561 s since 1904-01-01), "file name str"="D:\\Data\\Ultrasound\\LSCO\\LSCO22__130814c\\5_Cooling_2nd_try\\September_2014\\091614\\187.67800K_500_2500_2.10000V_0.00000T_Sep16-2014__15-12-41_001_091614.bin", "mod time(min)"=58228992.68333333, "file format"=enum."binary", "power(V)"=2.1, "Magn Field(T) "=0.0}, {"temperature"=187.365, "temperature str"="187.36500", "file path"=path "D:/Data/Ultrasound/LSCO/LSCO22__130814c/5_Cooling_2nd_try/September_2014/091614/187.36500K_500_2500_2.10000V_0.00000T_Sep16-2014__15-14-00_001_091614.bin", "last mod"=timestamp(3493739640 s since 1904-01-01), "file name str"="D:\\Data\\Ultrasound\\LSCO\\LSCO22__130814c\\5_Cooling_2nd_try\\September_2014\\091614\\187.36500K_500_2500_2.10000V_0.00000T_Sep16-2014__15-14-00_001_091614.bin", "mod time(min)"=58228994.0, "file format"=enum."binary", "power(V)"=2.1, "Magn Field(T) "=0.0}, {"temperature"=187.059, "temperature str"="187.05900", "file path"=path "D:/Data/Ultrasound/LSCO/LSCO22__130814c/5_Cooling_2nd_try/September_2014/091614/187.05900K_500_2500_2.10000V_0.00000T_Sep16-2014__15-15-20_001_091614.bin", "last mod"=timestamp(3493739720 s since 1904-01-01), "file name str"="D:\\Data\\Ultrasound\\LSCO\\LSCO22__130814c\\5_Cooling_2nd_try\\September_2014\\091614\\187.05900K_500_2500_2.10000V_0.00000T_Sep16-2014__15-15-20_001_091614.bin", "mod time(min)"=58228995.333333336, "file format"=enum."binary", "power(V)"=2.1, "Magn Field(T) "=0.0}, {"temperature"=186.735, "temperature str"="186.73500", "file path"=path "D:/Data/Ultrasound/LSCO/LSCO22__130814c/5_Cooling_2nd_try/September_2014/091614/186.73500K_500_2500_2.10000V_0.00000T_Sep16-2014__15-16-39_001_091614.bin", "last mod"=timestamp(3493739799 s since 1904-01-01), "file name str"="D:\\Data\\Ultrasound\\LSCO\\LSCO22__130814c\\5_Cooling_2nd_try\\September_2014\\091614\\186.73500K_500_2500_2.10000V_0.00000T_Sep16-2014__15-16-39_001_091614.bin", "mod time(min)"=58228996.65, "file format"=enum."binary", "power(V)"=2.1, "Magn Field(T) "=0.0}, {"temperature"=186.417, "temperature str"="186.41700", "file path"=path "D:/Data/Ultrasound/LSCO/LSCO22__130814c/5_Cooling_2nd_try/September_2014/091614/186.41700K_500_2500_2.10000V_0.00000T_Sep16-2014__15-17-58_001_091614.bin", "last mod"=timestamp(3493739878 s since 1904-01-01), "file name str"="D:\\Data\\Ultrasound\\LSCO\\LSCO22__130814c\\5_Cooling_2nd_try\\September_2014\\091614\\186.41700K_500_2500_2.10000V_0.00000T_Sep16-2014__15-17-58_001_091614.bin", "mod time(min)"=58228997.96666667, "file format"=enum."binary", "power(V)"=2.1, "Magn Field(T) "=0.0}, {"temperature"=186.086, "temperature str"="186.08600", "file path"=path "D:/Data/Ultrasound/LSCO/LSCO22__130814c/5_Cooling_2nd_try/September_2014/091614/186.08600K_500_2500_2.10000V_0.00000T_Sep16-2014__15-19-18_001_091614.bin", "last mod"=timestamp(3493739958 s since 1904-01-01), "file name str"="D:\\Data\\Ultrasound\\LSCO\\LSCO22__130814c\\5_Cooling_2nd_try\\September_2014\\091614\\186.08600K_500_2500_2.10000V_0.00000T_Sep16-2014__15-19-18_001_091614.bin", "mod time(min)"=58228999.3, "file format"=enum."binary", "power(V)"=2.1, "Magn Field(T) "=0.0}, {"temperature"=185.758, "temperature str"="185.75800", "file path"=path "D:/Data/Ultrasound/LSCO/LSCO22__130814c/5_Cooling_2nd_try/September_2014/091614/185.75800K_500_2500_2.10000V_0.00000T_Sep16-2014__15-20-37_001_091614.bin", "last mod"=timestamp(3493740037 s since 1904-01-01), "file name str"="D:\\Data\\Ultrasound\\LSCO\\LSCO22__130814c\\5_Cooling_2nd_try\\September_2014\\091614\\185.75800K_500_2500_2.10000V_0.00000T_Sep16-2014__15-20-37_001_091614.bin", "mod time(min)"=58229000.61666667, "file format"=enum."binary", "power(V)"=2.1, "Magn Field(T) "=0.0}, {"temperature"=185.416, "temperature str"="185.41600", "file path"=path "D:/Data/Ultrasound/LSCO/LSCO22__130814c/5_Cooling_2nd_try/September_2014/091614/185.41600K_500_2500_2.10000V_0.00000T_Sep16-2014__15-21-57_001_091614.bin", "last mod"=timestamp(3493740117 s since 1904-01-01), "file name str"="D:\\Data\\Ultrasound\\LSCO\\LSCO22__130814c\\5_Cooling_2nd_try\\September_2014\\091614\\185.41600K_500_2500_2.10000V_0.00000T_Sep16-2014__15-21-57_001_091614.bin", "mod time(min)"=58229001.95, "file format"=enum."binary", "power(V)"=2.1, "Magn Field(T) "=0.0}, {"temperature"=185.07, "temperature str"="185.07000", "file path"=path "D:/Data/Ultrasound/LSCO/LSCO22__130814c/5_Cooling_2nd_try/September_2014/091614/185.07000K_500_2500_2.10000V_0.00000T_Sep16-2014__15-23-16_001_091614.bin", "last mod"=timestamp(3493740196 s since 1904-01-01), "file name str"="D:\\Data\\Ultrasound\\LSCO\\LSCO22__130814c\\5_Cooling_2nd_try\\September_2014\\091614\\185.07000K_500_2500_2.10000V_0.00000T_Sep16-2014__15-23-16_001_091614.bin", "mod time(min)"=58229003.266666666, "file format"=enum."binary", "power(V)"=2.1, "Magn Field(T) "=0.0}, {"temperature"=184.744, "temperature str"="184.74400", "file path"=path "D:/Data/Ultrasound/LSCO/LSCO22__130814c/5_Cooling_2nd_try/September_2014/091614/184.74400K_500_2500_2.10000V_0.00000T_Sep16-2014__15-24-35_001_091614.bin", "last mod"=timestamp(3493740275 s since 1904-01-01), "file name str"="D:\\Data\\Ultrasound\\LSCO\\LSCO22__130814c\\5_Cooling_2nd_try\\September_2014\\091614\\184.74400K_500_2500_2.10000V_0.00000T_Sep16-2014__15-24-35_001_091614.bin", "mod time(min)"=58229004.583333336, "file format"=enum."binary", "power(V)"=2.1, "Magn Field(T) "=0.0}, {"temperature"=184.426, 
